vi "GetClimb_.vi"(8 "error in (no error)":errorcluster, 11 "Climber in":refnum<class "Climber.lvclass">) -> (0 "error out":errorcluster, 2 "Climb?":bool, 3 "Climber out":refnum<class "Climber.lvclass">)   [LabVIEW 2016, in "Climber.lvclass"]
uses:
  Climber.lvclass
  Climber.lvclass/Climber.ctl
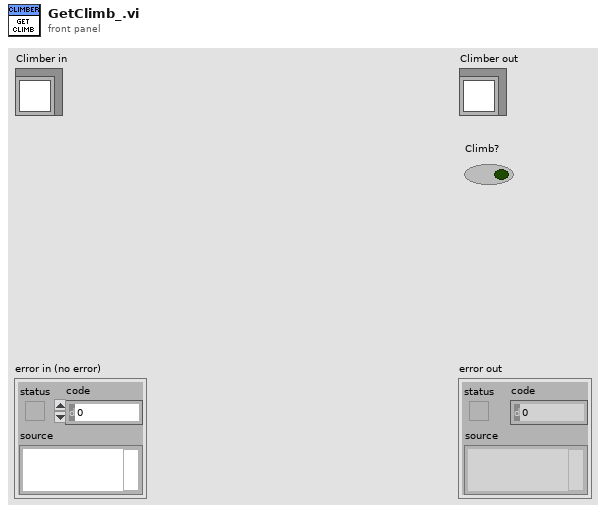
[diagram p1: front panel]
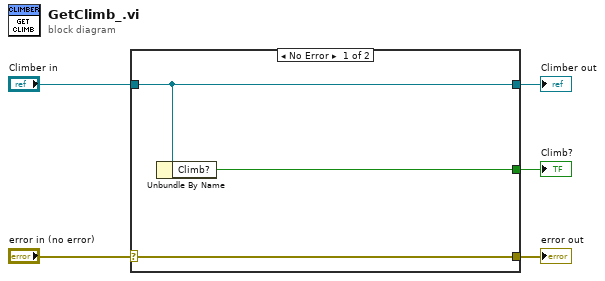
[diagram p0: block diagram]
diagram:
  n1 = case shown="No Error" "error in (no error)" {
    selector: "error in (no error)" -> [w8 w9]
    tunnel: [w8 w9] -> w4
    tunnel: [w7 w10] -> w2
    tunnel: "Climber in" -> [w7 w10]
    tunnel: [w6 _] -> w1
    frame No Error {
      n2 = Unbundle By Name(w7) -> ("Climb?"=w6:bool)
    }
    frame Error {
    }
  }
  "error out" <- w4
  "Climber out" <- w2
  "Climb?" <- w1
